vi "IMAQ forward movie.vi"(0 "Forwarded Phase":T1, 1 "n_grid":i32=400, 2 "Source Intensity (U16)":u16[][](array[numeric]), 5 "Forwarded Intensity":T1, 7 "error in (no error)":errorcluster, 9 "size_grid":dbl, 11 "lambda":dbl, 12 "Forward Distance":dbl, 13 "Source Phase (Float)":sgl[][](array[numeric]) format="%.2f") -> (15 "error out":errorcluster)   [LabVIEW 2012, in "LightPipes.lvlib"]
uses:
  LightPipes.lvlib
  <vilib>/vision/Image Controls.llb/IMAQ Image.ctl
panel:
  out "Forwarded Phase":T1(plugin-control)
  out "Forwared Int":T1(plugin-control)
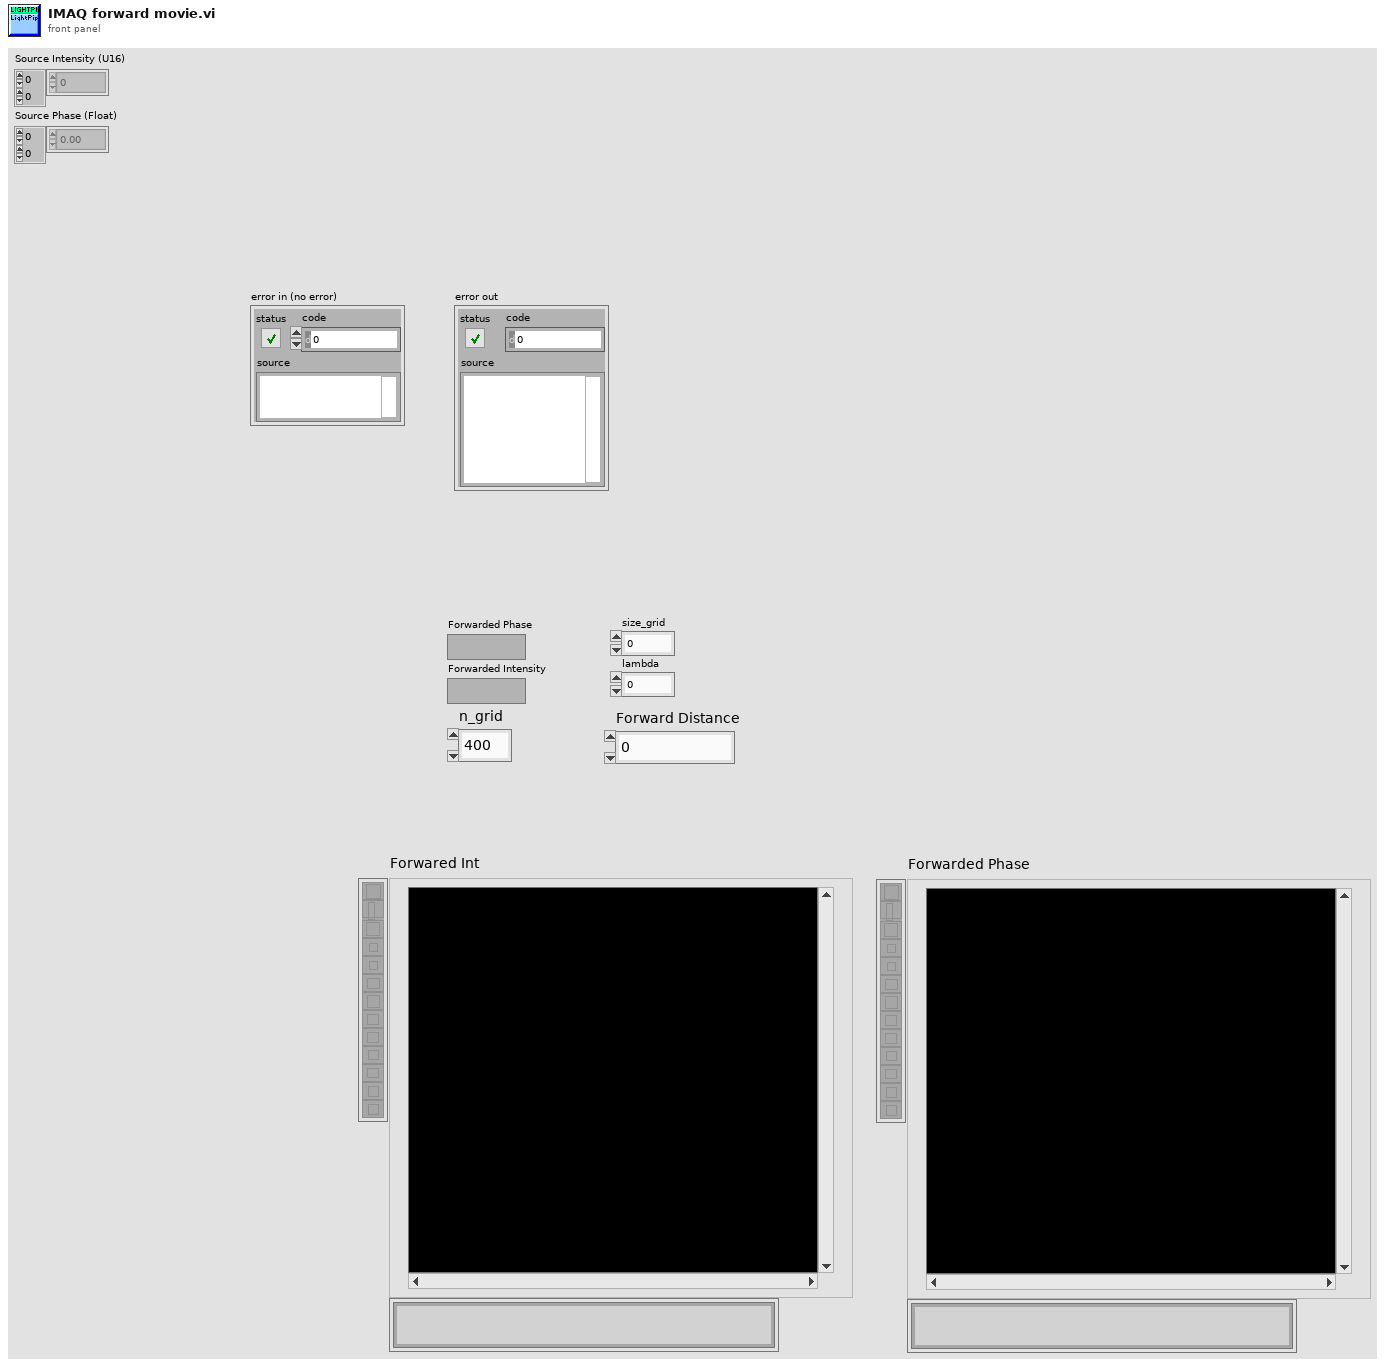
[diagram p1: front panel]
types:
  T1 = typedef "IMAQ Image.ctl" = refnum<image>
  T2 = cluster{"n_grid":i32, "@dummy control@":i8, "@dummy control@":i8, "@dummy control@":i8, "@dummy control@":i8, "size":dbl, "lambda":dbl, "int1":i32, "int2":i32, "int3":i32, "@dummy control@":i8, "@dummy control@":i8, "@dummy control@":i8, "@dummy control@":i8, "double1":dbl, "double2":dbl, "double3":dbl, "real":u32, "imaginary":u32}
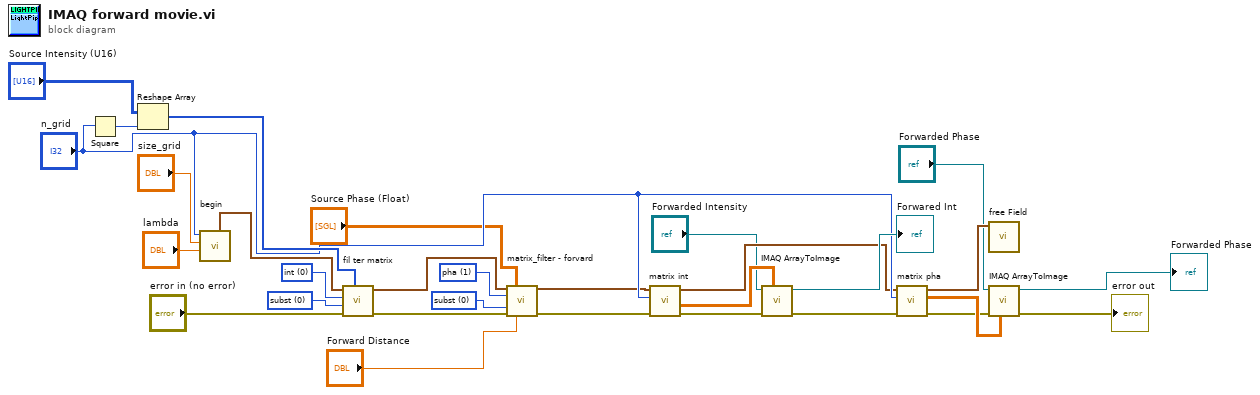
[diagram p0: block diagram]
diagram:
  w21 = i16 0 items=["subst", "mult"] ("multiplication/ substitution")
  w22 = i16 1 items=["int", "pha"] ("intensity / phase")
  w17 = i16 0 items=["int", "pha"] ("intensity / phase")
  w18 = i16 0 items=["subst", "mult"] ("multiplication/ substitution")
  n1 = Square(x="n_grid") -> (x^2=w26:i32)
  n2 = Reshape Array "Reshape Array"("Source Intensity (U16)", w26) -> (w27:u16[])
  n3 = call "begin.vi"("lambda"="lambda", "size_grid"="size_grid", "n_grid"="n_grid") -> ("field out"=w20:T2)  [unwired: 8 in]
  n4 = call "fil ter matrix.vi"("matrix"=w27, "error in (no error)"="error in (no error)", "multiplication/ substitution"=w18, "intensity / phase"=w17, "field"=w20) -> ("error out"=w2:errorcluster, "field out"=w19:T2)  [unwired: 4 in, 1 out]
  n5 = call "matrix_filter - forvard.vi"("field"=w19, "matrix in"="Source Phase (Float)", "intensity/phase"=w22, "multiplication/substitution"=w21, "error in (no error)"=w2, "forward distance"="Forward Distance") -> ("field out"=w16:T2, "error out"=w11:errorcluster)  [unwired: 8 in]
  n6 = call "matrix int.vi"("error in (no error)"=w11, "n_grid"="n_grid", "field"=w16) -> ("error out"=w9:errorcluster, "matrix out 2D"=w12:dbl[][], "field out"=w15:T2)  [unwired: 6 in]
  n7 = call "IMAQ ArrayToImage"("Image Pixels (U16)"=w12, "error in (no error)"=w9, "Image"="Forwarded Intensity") -> ("error out"=w7:errorcluster, "Image Out"=→"Forwared Int":T1)  [unwired: 7 in]
  n8 = call "matrix pha.vi"("error in (no error)"=w7, "n_grid"="n_grid", "field"=w15) -> ("error out"=w8:errorcluster, "matrix out 2D"=w13:dbl[][], "field out"=w30:T2)  [unwired: 6 in]
  n9 = call "free Field.vi"("field"=w30) -> ()  [unwired: 10 in, 1 out]
  n10 = call "IMAQ ArrayToImage"("Image Pixels (Float)"=w13, "error in (no error)"=w8, "Image"="Forwarded Phase") -> ("error out"=→"error out":errorcluster, "Image Out"=→"Forwarded Phase":T1)  [unwired: 7 in]
